vi "Teleop.vi"(10 "Match Info":T1={"Autonomous Elapsed Seconds"=0.0, "TeleOp Elapsed Seconds"=0.0, "Disabled Elapsed Seconds"=0.0, "Visited Autonomous"=FALSE, "Visited TeleOp"=FALSE, "Visited Disabled"=FALSE, "Autonomous Settings"={"Autonomous Style"=enum."Independent", "VI Refnum"=refnum}}, 11 "Call Context":T2) -> ()   [LabVIEW 2016]
doc: "This VI is called for each TeleOp packet received from the DS where the robot is not disabled. It is often used to read from the joysticks and update I/O or to update setpoints for timed control loops. It should complete and return within 20 milliseconds or it may miss DS packets."
uses:
  <vilib>/Rock Robotics/WPI/DriverStation/WPI_DriverStationDerivedRobotMode.ctl
  <vilib>/Rock Robotics/WPI/DriverStation/WPI_DriverStationMatch Info.ctl
  <vilib>/Rock Robotics/WPI/ThirdParty/CanMotor/TalonSRX/WPI_CANTalonSRX_APIFeedbackSelect.ctl
  <vilib>/Rock Robotics/WPI/ThirdParty/CanMotor/TalonSRX/WPI_CANTalonSRX_APIControlMode.ctl
  <vilib>/Rock Robotics/WPI/Utilities/WPI_GetSetVariantRefNum.vi
  <vilib>/Rock Robotics/Network Tables/NT Write Boolean Array.vi
  <vilib>/Rock Robotics/Network Tables/NT Write Numeric Array.vi
  <vilib>/Rock Robotics/Network Tables/NT Read Boolean.vi
  <vilib>/Rock Robotics/Network Tables/NT Read Number.vi
panel:
  out "Battery Voltage":dbl
  out "Current":dbl
  out "Encoder Position 2":dbl
  out "Encoder Position":dbl
  out "SensorPosRotations":dbl
  out "Motor output Plot":cluster{"Applied Throttle":dbl}(graph)
  out "Target RPM":dbl
  out "SensorRPM Velocity RPM":dbl
  out "Applied Output":dbl
  out "Speed Closed Loop Plots":cluster{dbl, "Sensor Velocity":dbl}(graph)
  in  "Enable":bool=TRUE
  in  "Reset":bool
  out "Table":string[][](table)
  out "Encoder Velocity":dbl
  out "Sample Slider 0":dbl(slide) scale=0.0..5.0
  out "Sample Boolean 1":bool
  out "Sample Boolean 0":bool
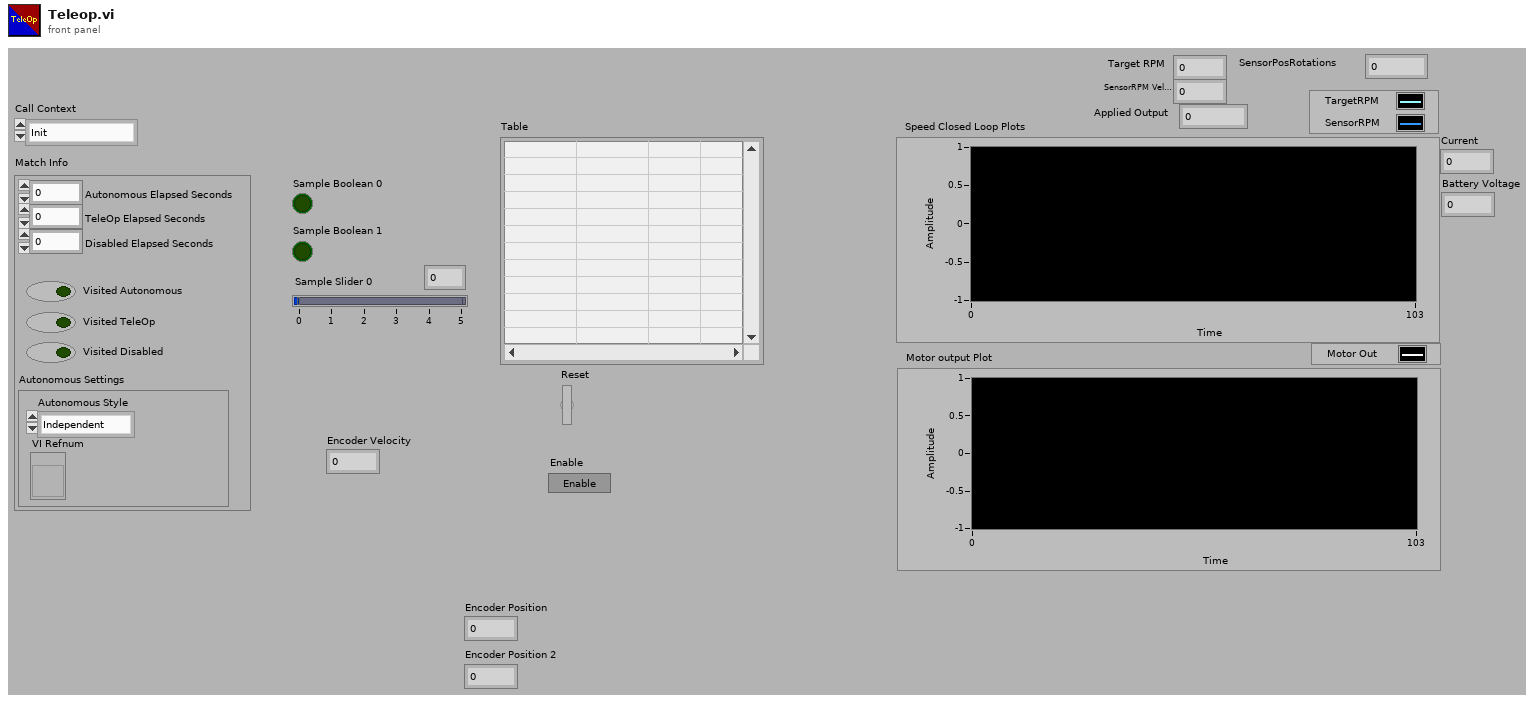
[diagram p1: front panel]
types:
  T1 = typedef "WPI_DriverStationMatch Info.ctl" = cluster{"Autonomous Elapsed Seconds":dbl, "TeleOp Elapsed Seconds":dbl, "Disabled Elapsed Seconds":dbl, "Visited Autonomous":bool, "Visited TeleOp":bool, "Visited Disabled":bool, "Autonomous Settings":cluster{"Autonomous Style":enum16{"Iterative", "Independent"}, "VI Refnum":refnum<vi>}}
  T2 = typedef "WPI_DriverStationDerivedRobotMode.ctl" = enum16{"Init", "Execute", "Stop"}
  T3 = typedef "WPI_CANTalonSRX_APIFeedbackSelect.ctl" = enum16{"Digital Quadrature Encoder", "Analog Potentiometer", "Analog Encoder", "Count on Quad-A (Rising-Edge)", "Count on Quad-A (Falling-Edge)", "CTR Magnetic Enc (Absolute)", "CTR Magnetic Enc (Relative)", "Pulse Width"}
  T4 = typedef "WPI_JoystickDevRef.ctl" = cluster{"Device":T5}
  T5 = typedef "WPI_JoystickDeviceEnum.ctl" = enum16{"USB 0", "USB 1", "USB 2", "USB 3", "USB 4", "USB 5"}
  T6 = typedef "WPI_RobotDriveDevRef.ctl" = cluster{"DevStatus":errorcluster, "Motors[]":T7[], "Square Inputs":bool, "Max Output":dbl}
  T7 = typedef "WPI_MotorControlDeviceRef.ctl" = cluster{"DeviceStatus":errorcluster, "Type":T8, "PWM":cluster{"PWM Channel":T9, "DeadBand":T10}, "CAN":cluster{"Device Number":u8, "SetOutput VI Ref":variant, "GetOutput VI Ref":variant, "Enable VI Ref":variant, "Disable VI Ref":variant, "Data":variant}, "Invert":bool}
  T8 = typedef "WPI_MotorControlType.ctl" = enum16{"PWM", "CAN"}
  T9 = typedef "FPGA_DIOPWMChannel.ctl" = enum8{"PWM 0", "PWM 1", "PWM 2", "PWM 3", "PWM 4", "PWM 5", "PWM 6", "PWM 7", "PWM 8", "PWM 9", "PWM MXP 0", "PWM MXP 1", "PWM MXP 2", "PWM MXP 3", "PWM MXP 4", "PWM MXP 5", "PWM MXP 6", "PWM MXP 7", "PWM MXP 8", "PWM MXP 9", "Invalid"}
  T10 = typedef "WPI_PWMDeadband.ctl" = cluster{"Name":string, "maxPositivePwm":i32, "minPositivePwm":i32, "centerPwm":i32, "maxNegativePwm":i32, "minNegativePwm":i32, "angularRange":u16}
  T11 = typedef "WPI_DigitalInputDevRef.ctl" = cluster{"DevStatus":errorcluster, "DIO Channel":T12}
  T12 = typedef "FPGA_DIOChannel.ctl" = enum8{"DIO 0", "DIO 1", "DIO 2", "DIO 3", "DIO 4", "DIO 5", "DIO 6", "DIO 7", "DIO 8", "DIO 9", "DIO MXP 0", "DIO MXP 1", "DIO MXP 2", "DIO MXP 3", "DIO MXP 4", "DIO MXP 5", "DIO MXP 6", "DIO MXP 7", "DIO MXP 8", "DIO MXP 9", "DIO MXP 10", "DIO MXP 11", "DIO MXP 12", "DIO MXP 13", "DIO MXP 14", "DIO MXP 15", "SPI Port CS1", "SPI Port CS2", "SPI Port CS3", "SPI Port MISO", "SPI Port MOSI", "Invalid"}
  T13 = typedef "WPI_CANTalonSRX_GlobalStatus.ctl" = cluster{"Applied Throttle":dbl, "Module Enabled":bool, "CAN Error":errorcluster, "Closed Loop Error":dbl, "Forward Limit Switch Closed":bool, "Reverse Limit Switch Closed":bool, "Sensor Position":dbl, "Sensor Velocity":dbl, "Current":dbl, "Sticky Fault - Over Temp":bool, "Sticky Fault - Under Voltage":bool, "Sticky Fault - Forward Limit":bool, "Sticky Fault - Reverse Limit":bool, "Sticky Fault - Forward Soft Limit":bool, "Sticky Fault - Reverse Soft Limit":bool, "Brake is Enabled":bool, "Encoder Position":dbl, "Encoder Velocity":dbl, "Encoder Index Count":dbl, "Encoder A Pin State":bool, "Encoder B Pin State":bool, "Encoder Index Pin State":bool, "Analog In":dbl, "Analog In Velocity":dbl, "Temperature (C)":dbl, "Battery Voltage":dbl, "Control 5 Is Supported":bool, "Current Profile Slot Select":dbl, "Pos Div 8":bool, "Vel Div 4":bool, "Pulse Width Position":i32, "Pulse Width Velocity":i32, "Pulse Width Rise To Rise (us)":i32, "Pulse Width Rise To Fall (us)":i32, "Mot Prof Active Is Under Run":bool, "Mot Prof Active Has Under Run":bool, "Mot Prof Active Is Last":bool, "Mot Prof Active Velocity Only":bool, "Mot Prof Active Is Valid":bool, "Mot Prof Buffer Is Full":bool, "Mot Prof Active Profile Slot Select":i32, "Mot Prof NextID":i32, "Mot Prof Count":i32, "Mot Prof Active Velocity":dbl, "Mot Prof Active Position":dbl, "Mot Prof Output Enable":i32, "UsageFrame":u32}
  T14 = typedef "WPI_CANTalonSRX_APIControlMode.ctl" = enum8{"Percent VBus", "Speed", "Position", "Slave", "Unchanged / Invalid", "Voltage Compensation", "Current", "Motion Profile", "Motion Magic"}
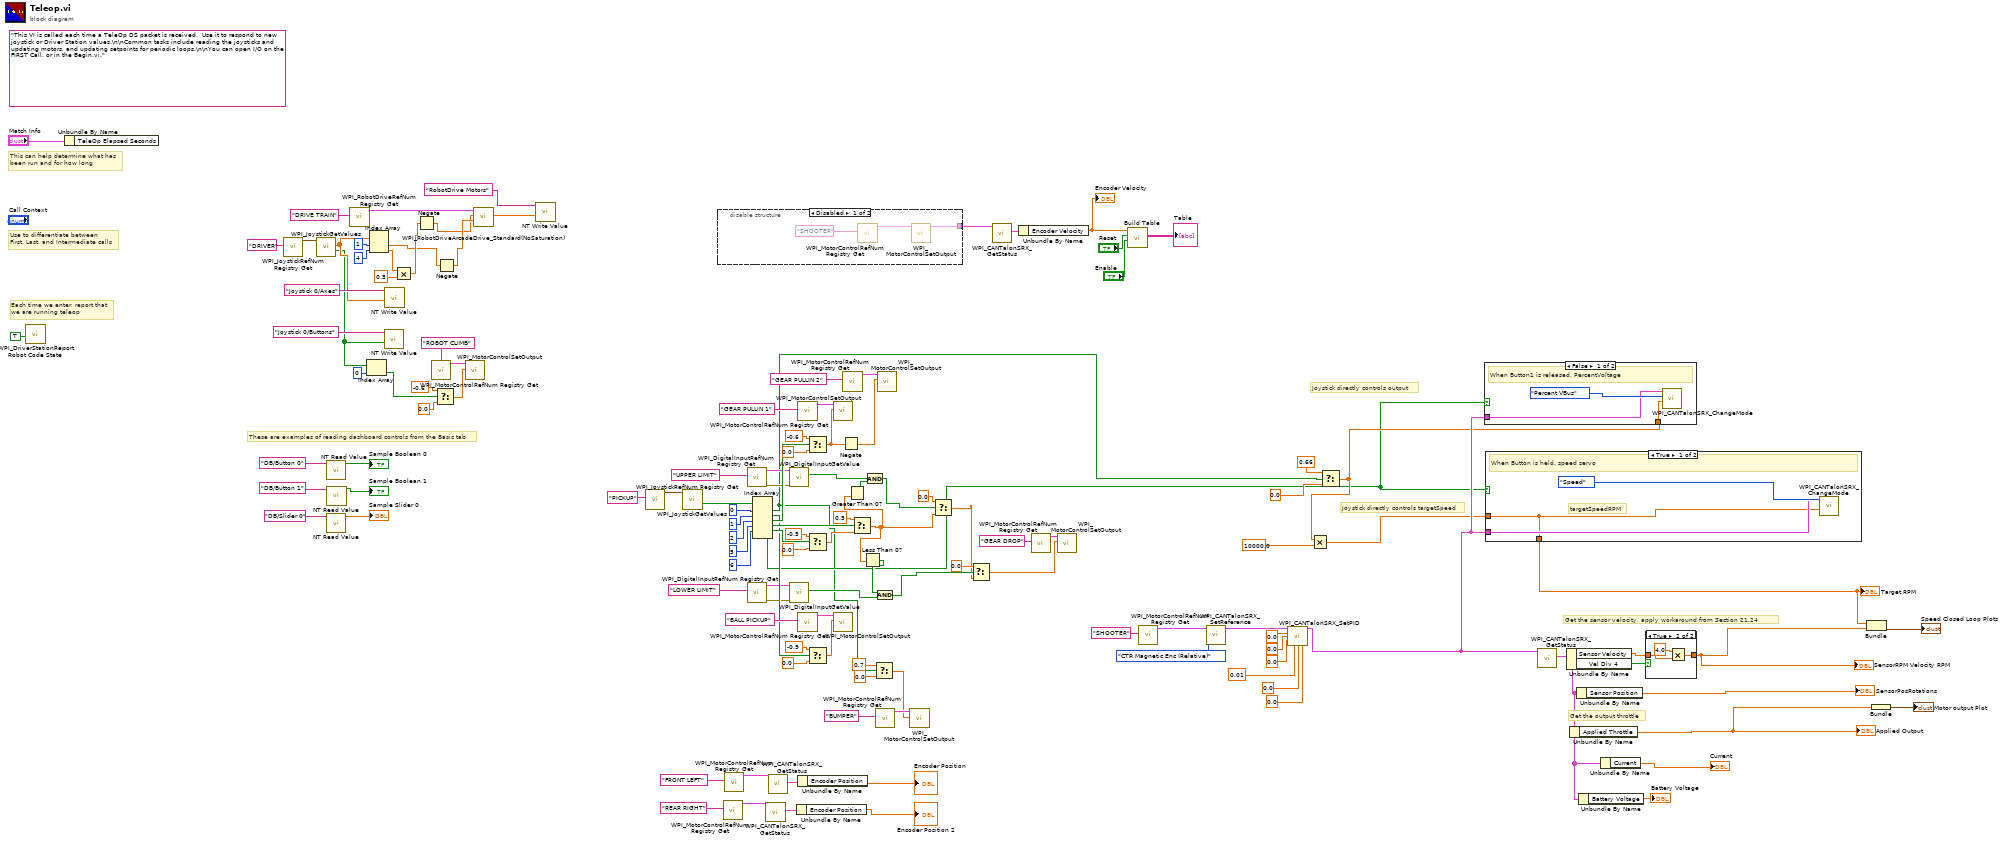
[diagram p0: block diagram]
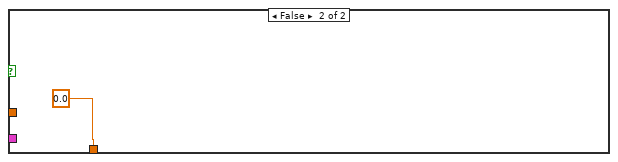
[diagram p4: hidden frame]
diagram:
  (unwired) "This VI is called each time a TeleOp DS packet is received.  Use it to respond to new joystick or Driver Station values.\n\nCommon tasks include reading the joysticks and updating motors, and updating setpoints for periodic loops.\n\nYou can open I/O on the FIRST Call, or in the Begin.vi."
  # "Get the output throttle"
  # "Get the sensor velocity, apply workaround from Section 21.24"
  # "Joystick directly controls targetSpeed"
  # "Joystick directly controls output"
  # "These are examples of reading dashboard controls from the Basic tab"
  # "Each time we enter, report that\nwe are running teleop"
  # "Use to differentiate between\nFirst, Last, and Intermediate calls"
  # "This can help determine what has\nbeen run and for how long"
  n1 = call <vilib>:"WPI_DriverStationReport Robot Code State.vi"("TeleOp"=TRUE ("Autonomous")) -> ()  [unwired: 10 in, 1 out]
  n2 = Unbundle By Name("Match Info") -> ()  [unwired: 1 out]
  n3 = call <vilib>:"WPI_JoystickRefNum Registry Get.vi"("refnum name"="DRIVER") -> ("JoystickDevRef"=w125:T4)  [unwired: 1 in, 9 out]
  n4 = call <vilib>:"WPI_JoystickGetValues.vi"("JoystickDevRef"=w125) -> ("Buttons"=w82:bool[], "Axes"=w121:dbl[])  [unwired: 6 in, 3 out]
  n5 = call-poly <vilib>:"NT Read Value.vi"("Name"="DB/Button 0" ("refnum name")) -> ("Boolean"=→"Sample Boolean 0":bool)  [unwired: 9 in, 1 out]
  n6 = call-poly <vilib>:"NT Read Value.vi"("Name"="DB/Slider 0" ("refnum name")) -> ("Numeric"=→"Sample Slider 0":dbl)  [unwired: 9 in, 1 out]
  n7 = call-poly <vilib>:"NT Read Value.vi"("Name"="DB/Button 1" ("refnum name")) -> ("Boolean"=→"Sample Boolean 1":bool)  [unwired: 9 in, 1 out]
  n8 = call <vilib>:"WPI_RobotDriveRefNum Registry Get.vi"("refnum name"="DRIVE TRAIN") -> ("RobotDriveDevRef"=w127:T6)  [unwired: 1 in, 9 out]
  n9 = Index Array(array=w82, index=0) -> (element=w78:bool)
  n10 = Index Array(array=w121, index #1=1 ("index"), index #2=4 ("index")) -> (element #1=w5:dbl, element #2=w70:dbl)
  n11 = call-poly <vilib>:"NT Write Value.vi"("Boolean Array"=w82, "Name"="Joystick 0/Buttons") -> ()  [unwired: 9 in, 1 out]
  n12 = call-poly <vilib>:"NT Write Value.vi"("Numeric Array"=w121, "Name"="Joystick 0/Axes") -> ()  [unwired: 9 in, 1 out]
  n13 = Multiply(x=w70, y=0.5) -> (x*y=w57:dbl)
  n14 = Negate(x=w57) -> (-x=w56:dbl)
  n15 = call <vilib>:"WPI_MotorControlRefNum Registry Get.vi"("refnum name"="ROBOT CLIMB") -> ("MotorControlDevRef"=w80:T7)  [unwired: 9 in, 1 out]
  n16 = Select(t=-0.6, s=w78, f=0.0) -> (s? t:f=w79:dbl)
  n17 = Negate(x=w5) -> (-x=w58:dbl)
  n18 = call <vilib>:"WPI_MotorControlSetOutput.vi"("Output"=w79, "MotorControlDevRef"=w80) -> ()  [unwired: 7 in, 3 out]
  n19 = call <vilib>:"WPI_RobotDriveArcadeDrive_Standard(NoSaturation).vi"("Y axis value"=w58, "X axis value"=w56, "RobotDriveDevRef"=w127) -> ("Motor Values"=w114:dbl[])  [unwired: 1 in, 7 out]
  n20 = call-poly <vilib>:"NT Write Value.vi"("Numeric Array"=w114, "Name"="RobotDrive Motors") -> ()  [unwired: 9 in, 1 out]
  n21 = call <vilib>:"WPI_JoystickRefNum Registry Get.vi"("refnum name"="PICKUP") -> ("JoystickDevRef"=w112:T4)  [unwired: 1 in, 9 out]
  n22 = call <vilib>:"WPI_JoystickGetValues.vi"("JoystickDevRef"=w112) -> ("Buttons"=w110:bool[])  [unwired: 6 in, 4 out]
  n23 = disable-structure shown="Disabled" {
    disable-tunnel: [w130 _] -> w74
    frame Disabled {
      n24 = call <vilib>:"WPI_MotorControlRefNum Registry Get.vi"("refnum name"="SHOOTER") -> ("MotorControlDevRef"=w131:T7)  [unwired: 9 in, 1 out]
      n25 = call <vilib>:"WPI_MotorControlSetOutput.vi"("MotorControlDevRef"=w131) -> ("MotorControlDevRef"=w130:T7)  [unwired: 8 in, 2 out]
    }
    frame Enabled {
    }
  }
  n26 = call <vilib>:"WPI_MotorControlRefNum Registry Get.vi"("refnum name"="REAR RIGHT") -> ("MotorControlDevRef"=w9:T7)  [unwired: 9 in, 1 out]
  n27 = call <vilib>:"WPI_MotorControlRefNum Registry Get.vi"("refnum name"="FRONT LEFT") -> ("MotorControlDevRef"=w10:T7)  [unwired: 9 in, 1 out]
  n28 = call <vilib>:"WPI_DigitalInputRefNum Registry Get.vi"("refnum name"="UPPER LIMIT") -> ("error out"=w64:errorcluster, "DigitalInputDevRef"=w63:T11)  [unwired: 9 in]
  n29 = call <vilib>:"WPI_DigitalInputRefNum Registry Get.vi"("refnum name"="LOWER LIMIT") -> ("error out"=w61:errorcluster, "DigitalInputDevRef"=w62:T11)  [unwired: 9 in]
  n30 = Index Array(array=w110, index #1=0 ("index"), index #2=1 ("index"), index #3=2 ("index"), index #4=5 ("index"), index #5=6 ("index")) -> (element #1=w16:bool, element #2=w85:bool, element #3=w92:bool, element #4=w91:bool, element #5=w90:bool, element #6=w19:bool)  [unwired: 1 in]
  n31 = call <vilib>:"WPI_CANTalonSRX_GetStatus.vi"("CAN Talon SRX Ref"=w9) -> ("Talon SRX Status"=w8:T13)  [unwired: 8 in, 2 out]
  n32 = call <vilib>:"WPI_CANTalonSRX_GetStatus.vi"("CAN Talon SRX Ref"=w10) -> ("Talon SRX Status"=w7:T13)  [unwired: 8 in, 2 out]
  n33 = call <vilib>:"WPI_DigitalInputGetValue.vi"("error in (no error)"=w64, "DigitalInputDevRef"=w63) -> ("Value"=w45:bool)  [unwired: 7 in, 2 out]
  n34 = call <vilib>:"WPI_DigitalInputGetValue.vi"("error in (no error)"=w61, "DigitalInputDevRef"=w62) -> ("Value"=w44:bool)  [unwired: 7 in, 2 out]
  n35 = Unbundle By Name(w8) -> ("Encoder Position"=→"Encoder Position 2":dbl)
  n36 = Unbundle By Name(w7) -> ("Encoder Position"=→"Encoder Position":dbl)
  n37 = call <vilib>:"WPI_MotorControlRefNum Registry Get.vi"("refnum name"="GEAR PULLIN 1") -> ("MotorControlDevRef"=w108:T7)  [unwired: 9 in, 1 out]
  n38 = call <vilib>:"WPI_MotorControlRefNum Registry Get.vi"("refnum name"="BALL PICKUP") -> ("MotorControlDevRef"=w89:T7)  [unwired: 9 in, 1 out]
  n39 = Select(t=-0.6, s=w92, f=0.0) -> (s? t:f=w102:dbl)
  n40 = Select(t=-0.5, s=w90, f=0.0) -> (s? t:f=w54:dbl)
  n41 = Select(t=-0.9, s=w85, f=0.0) -> (s? t:f=w87:dbl)
  n42 = call <vilib>:"WPI_MotorControlSetOutput.vi"("Output"=w102, "MotorControlDevRef"=w108) -> ()  [unwired: 7 in, 3 out]
  n43 = call <vilib>:"WPI_MotorControlSetOutput.vi"("Output"=w87, "MotorControlDevRef"=w89) -> ()  [unwired: 7 in, 3 out]
  n44 = Negate(x=w102) -> (-x=w101:dbl)
  n45 = call <vilib>:"WPI_MotorControlRefNum Registry Get.vi"("refnum name"="GEAR PULLIN 2") -> ("MotorControlDevRef"=w105:T7)  [unwired: 9 in, 1 out]
  n46 = Select(t=0.5, s=w91, f=w54) -> (s? t:f=w48:dbl)
  n47 = Greater Than 0?(x=w48) -> (x > 0?=w51:bool)
  n48 = Less Than 0?(x=w48) -> (x < 0?=w50:bool)
  n49 = And(x=w45, y=w51) -> (x .and. y?=w53:bool)
  n50 = Select(t=0.7, s=w16, f=0.0) -> (s? t:f=w13:dbl)
  n51 = And(x=w50, y=w44) -> (x .and. y?=w52:bool)
  n52 = call <vilib>:"WPI_MotorControlRefNum Registry Get.vi"("refnum name"="BUMPER") -> ("MotorControlDevRef"=w18:T7)  [unwired: 9 in, 1 out]
  n53 = call <vilib>:"WPI_MotorControlSetOutput.vi"("Output"=w101, "MotorControlDevRef"=w105) -> ()  [unwired: 7 in, 3 out]
  n54 = call <vilib>:"WPI_MotorControlSetOutput.vi"("Output"=w13, "MotorControlDevRef"=w18) -> ()  [unwired: 7 in, 3 out]
  n55 = Select(t=0.0, s=w53, f=w48) -> (s? t:f=w46:dbl)
  n56 = Select(t=0.0, s=w52, f=w46) -> (s? t:f=w55:dbl)
  n57 = call <vilib>:"WPI_CANTalonSRX_GetStatus.vi"("CAN Talon SRX Ref"=w74) -> ("Talon SRX Status"=w73:T13)  [unwired: 8 in, 2 out]
  n58 = Unbundle By Name(w73) -> ("Encoder Velocity"=w67:dbl)
  "Encoder Velocity" <- w67
  n59 = call <vilib>:"WPI_MotorControlRefNum Registry Get.vi"("refnum name"="GEAR DROP") -> ("MotorControlDevRef"=w99:T7)  [unwired: 9 in, 1 out]
  n60 = call <vilib>:"WPI_MotorControlSetOutput.vi"("Output"=w55, "MotorControlDevRef"=w99) -> ()  [unwired: 7 in, 3 out]
  n61 = call "Build Table"("Enable"="Enable", "Reset"="Reset", "Signals"=w67) -> ("Table"=→"Table":string[][])  [unwired: 2 in, 6 out]
  n62 = call <vilib>:"WPI_MotorControlRefNum Registry Get.vi"("refnum name"="SHOOTER") -> ("MotorControlDevRef"=w31:T7)  [unwired: 9 in, 1 out]
  n63 = call <vilib>:"WPI_CANTalonSRX_SetReference.vi"("Feedback Reference"=WPI_CANTalonSRX_APIFeedbackSelect."CTR Magnetic Enc (Relative)", "CAN Talon SRX Ref"=w31) -> ("CAN Talon SRX Ref"=w30:T7)  [unwired: 8 in, 1 out]
  n64 = call <vilib>:"WPI_CANTalonSRX_SetPID.vi"("CAN Talon SRX Ref"=w30, "P"=0.0, "I"=0.0, "D"=0.0, "F"=0.01, "I Zone"=0.0, "Ramp Rate"=0.0) -> ("CAN Talon SRX Ref"=w27:T7)  [unwired: 7 in, 1 out]
  n65 = Select(t=0.66 ("Output"), s=w16, f=0.0) -> (s? t:f=w21:dbl)
  n66 = Multiply(x=w21, y=10000.0) -> (x*y=w24:dbl)
  n67 = case shown="False" w19 {
    tunnel: w27 -> [w134 _]
    tunnel: w21 -> [w133 _]
    frame False {
      # "When Button1 is released, PercentVoltage"
      n68 = call <vilib>:"WPI_CANTalonSRX_ChangeMode.vi"("Output"=w133, "Control Mode"=WPI_CANTalonSRX_APIControlMode."Percent VBus", "CAN Talon SRX Ref"=w134) -> ()  [unwired: 7 in, 2 out]
    }
    frame True {
    }
  }
  n69 = case shown="True" w19 {
    tunnel: w24 -> [w136 _]
    tunnel: w27 -> [w137 _]
    tunnel: [w136 0.0 ("x")] -> w23
    frame True {
      # "targetSpeedRPM"
      # "When Button is held, speed servo"
      n70 = call <vilib>:"WPI_CANTalonSRX_ChangeMode.vi"("Output"=w136, "Control Mode"=WPI_CANTalonSRX_APIControlMode."Speed", "CAN Talon SRX Ref"=w137) -> ()  [unwired: 7 in, 2 out]
    }
    frame False {
    }
  }
  "Target RPM" <- w23
  n71 = call <vilib>:"WPI_CANTalonSRX_GetStatus.vi"("CAN Talon SRX Ref"=w27) -> ("Talon SRX Status"=w2:T13)  [unwired: 8 in, 2 out]
  n72 = Unbundle By Name(w2) -> ("Sensor Velocity"=w34:dbl, "Vel Div 4"=w33:bool)
  n73 = Unbundle By Name(w2) -> ("Applied Throttle"=w25:dbl)
  "Applied Output" <- w25
  n74 = Unbundle By Name(w2) -> ("Sensor Position"=→"SensorPosRotations":dbl)
  n75 = Unbundle By Name(w2) -> ("Battery Voltage"=→"Battery Voltage":dbl)
  n76 = Unbundle By Name(w2) -> ("Current"=→"Current":dbl)
  n77 = case shown="True" w33 {
    tunnel: [w140 w142] -> w32
    tunnel: w34 -> [w140 w141]
    frame False {
    }
    frame True {
      n78 = Multiply(x=4.0, y=w141) -> (x*y=w142:dbl)
    }
  }
  "SensorRPM Velocity RPM" <- w32
  n79 = Bundle("x"=w23, "Sensor Velocity"=w32) -> (→"Speed Closed Loop Plots":cluster{"x":dbl, "Sensor Velocity":dbl})  [unwired: 1 in]
  n80 = Bundle("Applied Throttle"=w25) -> (→"Motor output Plot":cluster{"Applied Throttle":dbl})  [unwired: 1 in]
